vi "Get Channels from Line.vi"(11 "Line":T1) -> (3 "Channels":refnum<class "TBM channel.lvclass">[](array[class]))   [LabVIEW 2018, in "Add Module configuration.lvclass"]
doc: "Returns an array of channels for a single line."
uses:
  Add Module configuration.lvclass
  <vilib>/NI/Tag Bus Module Framework/channel/TBM channel.lvclass
  Line.ctl
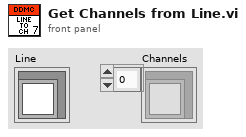
[diagram p1: front panel]
types:
  T1 = typedef "Add Module configuration.lvclass/Line.ctl" = cluster{"channel":refnum<class "TBM channel.lvclass">}
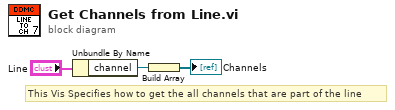
[diagram p0: block diagram]
diagram:
  # "This Vis Specifies how to get the all channels that are part of the line"
  n1 = Unbundle By Name("Line") -> ("channel"=w1:refnum<class "TBM channel.lvclass">)
  n2 = Build Array(w1) -> (→"Channels":refnum<class "TBM channel.lvclass">[])
